vi "AB_Create_Default_App_Destinations.vi"(5 "preserve hierarchy (T)":bool=TRUE, 7 "internal dir name":string, 8 "error in (no error)":errorcluster, 9 "SupportDirectory":string, 10 "App Name":string, 11 "App Destination Path":path) -> (0 "error out":errorcluster, 3 "default app dests":refnum<class "AB_Destination.lvclass">[](array[class]))   [LabVIEW 2020]
uses:
  <vilib>/AppBuilder/AB_Classes/Destination/AB_Destination.lvclass
  <vilib>/AppBuilder/AB_Classes/Destination/Dest_Application/AB_Dest_App.lvclass
  <vilib>/AppBuilder/AB_Classes/Destination/Dest_LegacyApplication/AB_Dest_LegacyApp.lvclass
  <vilib>/AppBuilder/AB_Classes/Destination/AB_Destination.ctl
  e:/builds/penguin/labview/branches/2020/dev/dist/vi.lib/AppBuilder/AB_Classes/Destination/AB_Destination.lvclass
  e:/builds/penguin/labview/branches/2020/dev/dist/vi.lib/AppBuilder/AB_Classes/Destination/Dest_Application/AB_Dest_App.lvclass
  e:/builds/penguin/labview/branches/2020/dev/dist/vi.lib/AppBuilder/AB_Classes/Destination/Dest_LLB/AB_Dest_LLB.lvclass
  e:/builds/penguin/labview/branches/2020/dev/dist/vi.lib/AppBuilder/AB_Classes/Destination/Dest_LegacyApplication/AB_Dest_LegacyApp.lvclass
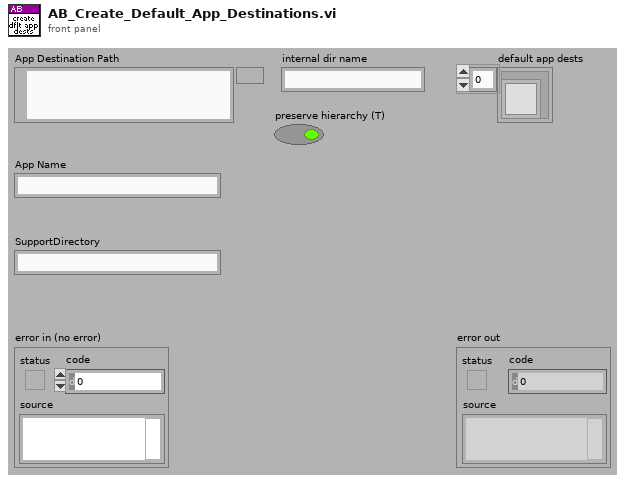
[diagram p1: front panel]
types:
  T1 = typedef "AB_Destination.ctl" = cluster{"destName":string, "path":path, "libraryName":string, "preserveHierarchy":bool, "eng_inBuild":bool, "eng_libraryReference":refnum<vi>, "eng_restictAddToNewLibrary":bool}
  T2 = enum32{"invalid OS target", "Mac OS", "Windows 3.1", "Windows 95/NT", "Solaris 1", "Solaris 2", "HP-UX", "PowerMAX", "Linux", "Irix", "Rhapsody", "BeOS", "AIX", "OSF1", "VxWorks", "PharLap", "Carbon", "RTX", "Windows x64", "Linux x64", "Mac OS X x64"}
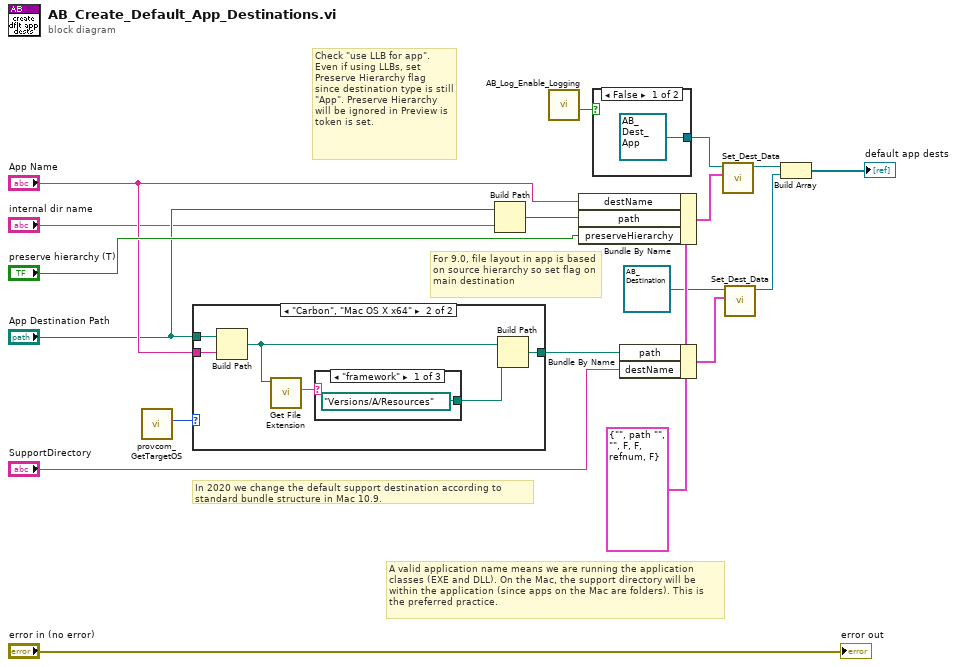
[diagram p0: block diagram]
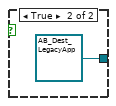
[diagram p2: hidden frame]
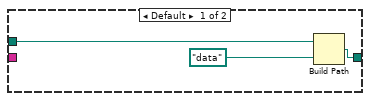
[diagram p3: hidden frame]
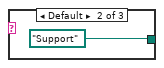
[diagram p4: hidden frame]
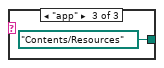
[diagram p5: hidden frame]
diagram:
  w18 = T1 {"destName"="", "path"=path "", "libraryName"="", "preserveHierarchy"=FALSE, "eng_inBuild"=FALSE, "eng_libraryReference"=refnum, "eng_restictAddToNewLibrary"=FALSE} ("destName")
  # "In 2020 we change the default support destination according to standard bundle structure in Mac 10.9."
  # "For 9.0, file layout in app is based on source hierarchy so set flag on main destination"
  # "Check \"use LLB for app\".\nEven if using LLBs, set Preserve Hierarchy flag  since destination type is still \"App\". Preserve Hierarchy will be ignored in Preview is token is set."
  # "A valid application name means we are running the application classes (EXE and DLL). On the Mac, the support directory will be within the application (since apps on the Mac are folders). This is the preferred practice."
  n1 = call <resource>:"provcom_GetTargetOS.vi"() -> ("App.TargetOS"=w12:T2)  [unwired: 11 out]
  n2 = case shown="\"Carbon\", \"Mac OS X x64\"" w12 {
    tunnel: "App Destination Path" -> [w20 w26]
    tunnel: [w19 w25] -> w14
    tunnel: "App Name" -> [_ w24]
    frame Default {
      n3 = Build Path(base path=w20, name or relative path=path "data") -> (appended path=w19:path)
    }
    frame "Carbon", "Mac OS X x64" {
      n4 = Build Path(base path=w26, name or relative path=w24) -> (appended path=w23:path)
      n5 = call <vilib>:"Get File Extension.vi"("file"=w23) -> ("lowercase file extension"=w22:string)  [unwired: 6 in, 4 out]
      n6 = case shown="\"framework\"" w22 {
        tunnel: [path "Versions/A/Resources" ("name or relative path") path "Support" ("name or relative path") path "Contents/Resources" ("name or relative path")] -> w27
        frame "framework" {
        }
        frame Default {
        }
        frame "app" {
        }
      }
      n7 = Build Path(base path=w23, name or relative path=w27) -> (appended path=w25:path)
    }
  }
  n8 = Build Path(base path="App Destination Path", name or relative path="internal dir name") -> (appended path=w6:path)
  n9 = call <vilib>:"AB_Log_Enable_Logging.vi"() -> ("use LLB for app"=w16:bool)  [unwired: 2 in, 9 out]
  n10 = Bundle By Name(cluster=w18, "destName"="App Name", "path"=w6, "preserveHierarchy"="preserve hierarchy (T)") -> (w7:T1)
  n11 = case shown="False" w16 {
    tunnel: [refnum<class "AB_Dest_App.lvclass"> refnum ("AB_Dest_App.lvclass") refnum<class "AB_Dest_LegacyApp.lvclass"> refnum ("AB_Dest_LegacyApp.lvclass")] -> w4
    frame False {
    }
    frame True {
    }
  }
  n12 = Bundle By Name(cluster=w18, "path"=w14, "destName"="SupportDirectory") -> (w10:T1)
  n13 = call <vilib>:"Set_Dest_Data.vi"("destName"=w7, "Class in"=w4) -> ("Class out"=w5:refnum<class "AB_Destination.lvclass">)  [unwired: 1 in, 8 out]
  n14 = call <vilib>:"Set_Dest_Data.vi"("destName"=w10, "Class in"=refnum<class "AB_Destination.lvclass"> refnum ("AB_Destination.lvclass")) -> ("Class out"=w9:refnum<class "AB_Destination.lvclass">)  [unwired: 1 in, 8 out]
  n15 = Build Array(w5, w9) -> (→"default app dests":refnum<class "AB_Destination.lvclass">[])
  "error out" <- "error in (no error)"
